vi "Query Slew Rate.vi"   [LabVIEW 2012, in "NH Research Regenerative Test Series.lvlib"]
doc: "Returns the slew rate set for all programmed changes in the output of the module."
uses:
  <instrlib>/NH Research Regenerative Test Series/NH Research Regenerative Test Series.lvlib
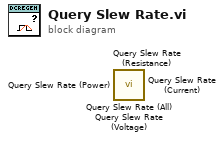
[diagram p0: block diagram]
diagram:
  n1 = call <instrlib>:"Query Slew Rate (All).vi"() -> ()  [unwired: 10 in, 6 out]
  n2 = call <instrlib>:"Query Slew Rate (Resistance).vi"() -> ()  [unwired: 13 in, 3 out]
  n3 = call <instrlib>:"Query Slew Rate (Power).vi"() -> ()  [unwired: 13 in, 3 out]
  n4 = call <instrlib>:"Query Slew Rate (Current).vi"() -> ()  [unwired: 13 in, 3 out]
  n5 = call <instrlib>:"Query Slew Rate (Voltage).vi"() -> ()  [unwired: 13 in, 3 out]
